vi "Perform Action.vi"(8 "error in (no error)":errorcluster, 10 "Input":variant, 11 "Read All CFG in":refnum<class "Read All CFG.lvclass">) -> (0 "error out":errorcluster, 2 "Output":variant, 3 "Read All CFG out":refnum<class "Read All CFG.lvclass">)   [LabVIEW 2023, in "NEO480HTA.lvlib" / "Read All CFG.lvclass"]
uses:
  Read All CFG.lvclass
  Read All CFG.lvclass/Read All CFG.ctl
  <vilib>/ErrorRing/Error Ring.xnode
  <vilib>/xnet/xnet.llb/XNET Read (Frame CAN).vi
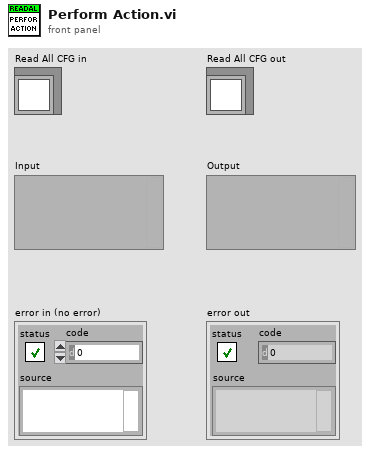
[diagram p1: front panel]
types:
  T1 = enum16{"Default", "Dew Point", "Pressure", "Temperature", "Sensor Status", "Dew Point Raw", "Absolute Humidity", "C H20"}
  T2 = typedef "XNET Frame CAN.ctl" = cluster{"timestamp":timestamp, "payload":u8[], "identifier":u32, "type":T3, "extended?":bool, "echo?":bool}
  T3 = typedef "XNET Frame Type CAN.ctl" = u8
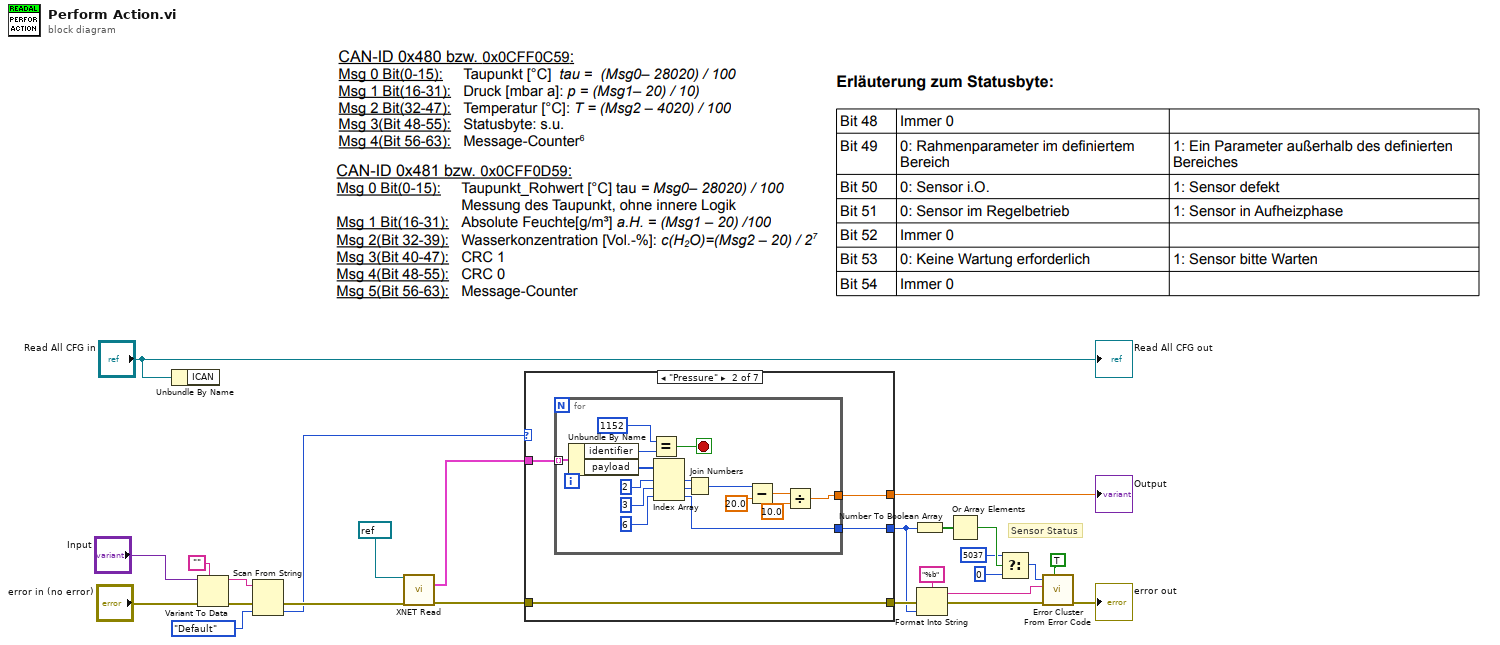
[diagram p0: block diagram]
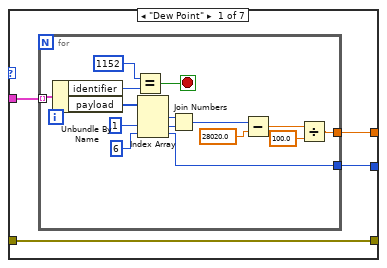
[diagram p2: hidden frame]
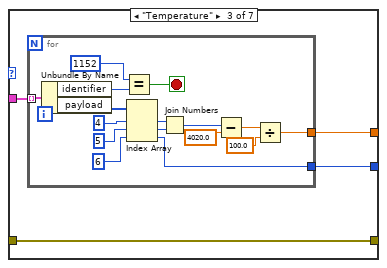
[diagram p3: hidden frame]
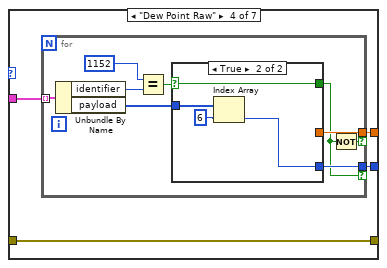
[diagram p4: hidden frame]
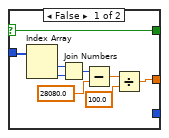
[diagram p5: hidden frame]
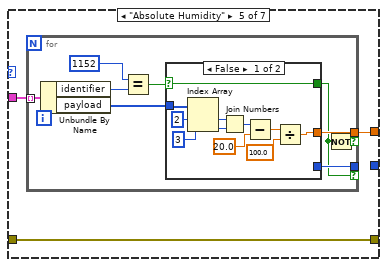
[diagram p6: hidden frame]
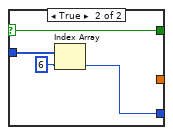
[diagram p7: hidden frame]
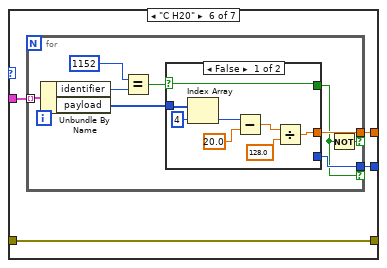
[diagram p8: hidden frame]
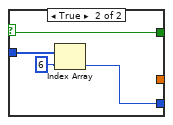
[diagram p9: hidden frame]
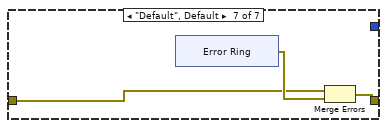
[diagram p10: hidden frame]
diagram:
  # "Sensor Status"
  n1 = Unbundle By Name("Read All CFG in") -> ()  [unwired: 1 out]
  n2 = Variant To Data(error in="error in (no error)", type="" ("Empty String Constant"), Variant="Input") -> (data=w18:string, error out=w24:errorcluster)
  n3 = Scan From String(input string=w18, error in=w24, default 1=T1."Default") -> (error out=w20:errorcluster, output 1=w3:T1)  [unwired: 2 in, 2 out]
  n4 = call-poly <vilib>:"XNET Read.vi"("session in"=refnum<k21> refnum, "error in (no error)"=w20) -> ("data"=w17:T2[], "error out"=w21:errorcluster)  [unwired: 12 out]
  n5 = case shown="\"Pressure\"" w3 {
    tunnel: w21 -> [w26 w46 w65 w86 w111 w138 w164]
    tunnel: [w26 w46 w65 w86 w111 w138 w163] -> w6
    tunnel: w17 -> [w29 w48 w68 w88 w113 w141 _]
    tunnel: [w28 w47 w67 w85 w112 w139 _] -> w16
    tunnel: [w27 w45 w66 w87 _ w140 _] -> w4
    frame "Dew Point" {
      n6 = for {
        tunnel: w29 -> [w44] mode=indexing
        tunnel: [w35] -> w28
        tunnel: [w31] -> w27
        stop <- w34 stop-if-true
        n7 = Unbundle By Name(w44) -> ("identifier"=w43:u32, "payload"=w39:u8[])
        n8 = Equal?(x=u32 1152, y=w43) -> (x = y?=w34:bool)
        n9 = Index Array(array=w39, index #2=1 ("index"), index #3=6 ("index")) -> (element #1=w38:u8, element #2=w37:u8, element #3=w31:u8)  [unwired: 1 in]
        n10 = Join Numbers(hi=w38, lo=w37) -> ((hi.lo)=w36:u16)
        n11 = Subtract(x=w36, y=28020.0) -> (x-y=w40:dbl)
        n12 = Divide(x=w40, y=100.0) -> (x/y=w35:dbl)
      }
    }
    frame "Pressure" {
      n13 = for {
        tunnel: w48 -> [w64] mode=indexing
        tunnel: [w53] -> w47
        tunnel: [w49] -> w45
        stop <- w60 stop-if-true
        n14 = Unbundle By Name(w64) -> ("identifier"=w63:u32, "payload"=w61:u8[])
        n15 = Equal?(x=u32 1152, y=w63) -> (x = y?=w60:bool)
        n16 = Index Array(array=w61, index #1=2 ("index"), index #2=3 ("index"), index #3=6 ("index")) -> (element #1=w56:u8, element #2=w55:u8, element #3=w49:u8)
        n17 = Join Numbers(hi=w56, lo=w55) -> ((hi.lo)=w54:u16)
        n18 = Subtract(x=w54, y=20.0) -> (x-y=w57:dbl)
        n19 = Divide(x=w57, y=10.0) -> (x/y=w53:dbl)
      }
    }
    frame "Temperature" {
      n20 = for {
        tunnel: w68 -> [w84] mode=indexing
        tunnel: [w74] -> w67
        tunnel: [w70] -> w66
        stop <- w80 stop-if-true
        n21 = Unbundle By Name(w84) -> ("identifier"=w83:u32, "payload"=w81:u8[])
        n22 = Equal?(x=u32 1152, y=w83) -> (x = y?=w80:bool)
        n23 = Index Array(array=w81, index #1=4 ("index"), index #2=5 ("index"), index #3=6 ("index")) -> (element #1=w77:u8, element #2=w76:u8, element #3=w70:u8)
        n24 = Join Numbers(hi=w77, lo=w76) -> ((hi.lo)=w75:u16)
        n25 = Subtract(x=w75, y=4020.0) -> (x-y=w78:dbl)
        n26 = Divide(x=w78, y=100.0) -> (x/y=w74:dbl)
      }
    }
    frame "Dew Point Raw" {
      n27 = for {
        tunnel: w88 -> [w97] mode=indexing
        tunnel: [w92] -> w87 if=w90
        tunnel: [w91] -> w85 if=w89
        n28 = Unbundle By Name(w97) -> ("identifier"=w96:u32, "payload"=w94:u8[])
        n29 = Equal?(x=u32 1152, y=w96) -> (x = y?=w93:bool)
        n30 = case shown="True" w93 {
          selector: w93 -> [w98 w107]
          tunnel: w94 -> [w106 w110]
          tunnel: [_ w108] -> w92
          tunnel: [w99 _] -> w91
          tunnel: [w98 w107] -> w90
          frame False {
            n31 = Index Array(array=w106) -> (element #1=w105:u8, element #2=w104:u8)  [unwired: 2 in]
            n32 = Join Numbers(hi=w105, lo=w104) -> ((hi.lo)=w103:u16)
            n33 = Subtract(x=w103, y=28080.0) -> (x-y=w101:dbl)
            n34 = Divide(x=w101, y=100.0) -> (x/y=w99:dbl)
          }
          frame True {
            n35 = Index Array(array=w110, index=6) -> (element=w108:u8)
          }
        }
        n36 = Not(x=w90) -> (.not. x?=w89:bool)
      }
    }
    frame "Absolute Humidity" {
      n37 = for {
        tunnel: w113 -> [w122] mode=indexing
        tunnel: [w117] -> _ if=w114
        tunnel: [w116] -> w112 if=w115
        n38 = Unbundle By Name(w122) -> ("identifier"=w121:u32, "payload"=w119:u8[])
        n39 = Equal?(x=u32 1152, y=w121) -> (x = y?=w118:bool)
        n40 = case shown="False" w118 {
          selector: w118 -> [w123 w134]
          tunnel: w119 -> [w133 w137]
          tunnel: [_ w135] -> w117
          tunnel: [w126 _] -> w116
          tunnel: [w123 w134] -> w114
          frame False {
            n41 = Index Array(array=w133, index #1=2 ("index"), index #2=3 ("index")) -> (element #1=w132:u8, element #2=w131:u8)
            n42 = Join Numbers(hi=w132, lo=w131) -> ((hi.lo)=w130:u16)
            n43 = Subtract(x=w130, y=20.0) -> (x-y=w128:dbl)
            n44 = Divide(x=w128, y=100.0) -> (x/y=w126:dbl)
          }
          frame True {
            n45 = Index Array(array=w137, index=6) -> (element=w135:u8)
          }
        }
        n46 = Not(x=w114) -> (.not. x?=w115:bool)
      }
    }
    frame "C H20" {
      n47 = for {
        tunnel: w141 -> [w150] mode=indexing
        tunnel: [w146] -> w140 if=w143
        tunnel: [w145] -> w139 if=w142
        n48 = Unbundle By Name(w150) -> ("identifier"=w149:u32, "payload"=w147:u8[])
        n49 = Equal?(x=u32 1152, y=w149) -> (x = y?=w144:bool)
        n50 = case shown="False" w144 {
          selector: w144 -> [w151 w159]
          tunnel: w147 -> [w158 w162]
          tunnel: [_ w160] -> w146
          tunnel: [w154 _] -> w145
          tunnel: [w151 w159] -> w143
          frame False {
            n51 = Index Array(array=w158, index=4) -> (element=w152:u8)
            n52 = Subtract(x=w152, y=20.0) -> (x-y=w156:dbl)
            n53 = Divide(x=w156, y=128.0) -> (x/y=w154:dbl)
          }
          frame True {
            n54 = Index Array(array=w162, index=6) -> (element=w160:u8)
          }
        }
        n55 = Not(x=w143) -> (.not. x?=w142:bool)
      }
    }
    frame "Default", Default {
      n56 = xnode "Error Ring"() -> ("error out"=w165:errorcluster)
      n57 = Merge Errors(w164, w165) -> (w163:errorcluster)
    }
  }
  "Output" <- w16
  n58 = Number To Boolean Array(number=w4) -> (Boolean array=w12:bool[])
  n59 = Format Into String(format string="%b", error in=w6, w4) -> (resulting string=w13:string, error out=w14:errorcluster)  [unwired: 1 in]
  n60 = Or Array Elements(Boolean array=w12) -> (logical OR=w11:bool)
  n61 = Select(t=5037, s=w11, f=0) -> (s? t:f=w15:i32)
  n62 = call <vilib>:"Error Cluster From Error Code.vi"("show call chain? (False)"=TRUE, "error in (no error)"=w14, "error message (\"\")"=w13, "error code (0)"=w15) -> ("error out"=→"error out":errorcluster)  [unwired: 5 in]
  "Read All CFG out" <- "Read All CFG in"
